vi "SRV_PM_Is Header Complete.vi"(0 "Packet Data":u8[](array[numeric]) format="%.0x", 11 "error in (no error)":errorcluster, 12 "Gen Err? (T)":bool=TRUE) -> (4 "Packet Data dup":u8[](array[numeric]) format="%.0x", 8 "Header OK?":bool, 15 "error out":errorcluster)   [LabVIEW 2014]
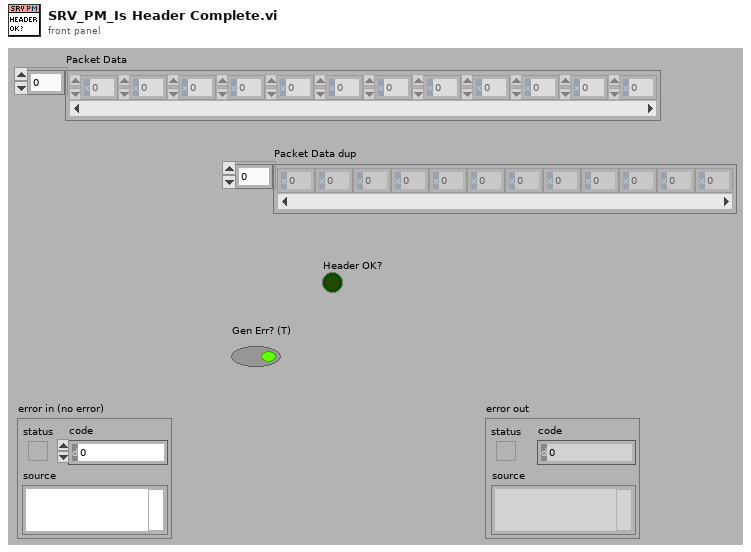
[diagram p1: front panel]
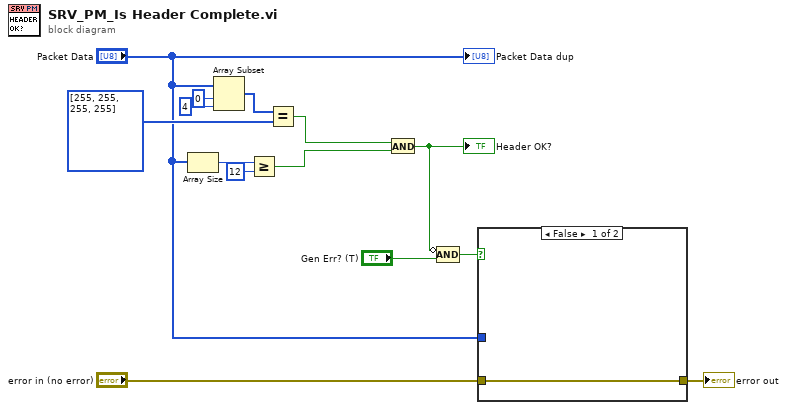
[diagram p0: block diagram]
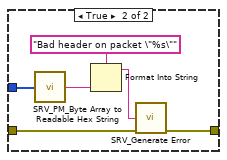
[diagram p2: hidden frame]
diagram:
  n1 = Array Size(array="Packet Data") -> (size(s)=w14:i32)
  n2 = Array Subset(array="Packet Data", index=0, length=4) -> (w10:u8[])
  n3 = Greater Or Equal?(x=w14, y=12) -> (x >= y?=w7:bool)
  n4 = Equal?(x=w10, y=u8[] [255, 255, 255, 255] ("subarray")) -> (x = y?=w8:bool)
  n5 = And(x=w8, y=w7) -> (x .and. y?=w4:bool)
  "Header OK?" <- w4
  n6 = Compound Arithmetic op=AND(invert w4, "Gen Err? (T)") -> (w5:bool)
  n7 = case shown="False" w5 {
    tunnel: "Packet Data" -> [_ w18]
    tunnel: "error in (no error)" -> [w15 w17]
    tunnel: [w15 w16] -> w1
    frame False {
    }
    frame True {
      n8 = call "SRV_PM_Byte Array to Readable Hex String.vi"("Byte Array"=w18) -> ("Readable Hex String"=w20:string)  [unwired: 14 in]
      n9 = Format Into String(format string="Bad header on packet \"%s\"" ("Message"), w20) -> (resulting string=w19:string)  [unwired: 2 in, 1 out]
      n10 = call "SRV_Generate Error.vi"("Message"=w19, "error in (no error)"=w17) -> ("error out"=w16:errorcluster)  [unwired: 13 in]
    }
  }
  "error out" <- w1
  "Packet Data dup" <- "Packet Data"
